vi "preprocess_pwm.vi"(1 "input":dbl) -> (0 "output":dbl[](array[numeric]))   [LabVIEW 2021]
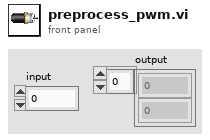
[diagram p1: front panel]
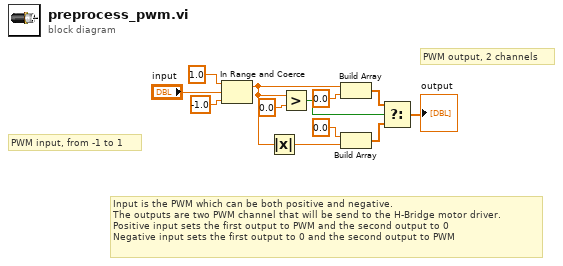
[diagram p0: block diagram]
diagram:
  # "Input is the PWM which can be both positive and negative.\nThe outputs are two PWM channel that will be send to the H-Bridge motor driver.\nPositive input sets the first output to PWM and the second output to 0\nNegative input sets the first output to 0 and the second output to PWM"
  # "PWM output, 2 channels"
  # "PWM input, from -1 to 1"
  n1 = In Range and Coerce(upper limit=1.0, x="input", lower limit=-1.0) -> (coerced(x)=w1:dbl)  [unwired: 1 out]
  n2 = Absolute Value(x=w1) -> (abs(x)=w2:dbl)
  n3 = Greater?(x=w1, y=0.0) -> (0:w12:bool)
  n4 = Build Array(w1, 0.0 ("element")) -> (w8:dbl[])
  n5 = Build Array(0.0 ("element"), w2) -> (w7:dbl[])
  n6 = Select(t=w8, s=w12, f=w7) -> (s? t:f=→"output":dbl[])
